vi "1553 Address Based Handles to Execution Unit Address Handles.vi"(8 "error in":errorcluster, 11 "1553 address based channel handles":T1[](array[typedef]) {"acyclic frame trigger handles"."handle" format="%.0x"; "start stop handles"."stop handle" format="%.0x"; "start stop handles"."start handle" format="%.0x"}) -> (0 "error out":errorcluster, 3 "address based channels":T4[](array[typedef]) format="%.0x")   [LabVIEW 2020, in "Ballard MIL-STD-1553 Engine.lvlib" / "Implementation.lvlib" / "Address Based Execution Unit.lvclass"]
uses:
  Address Based Execution Unit.lvclass
  <vilib>/NI VeriStand/Custom Device API/Custom Device Item Ref.ctl
  <vilib>/NI VeriStand/Custom Device API/Custom Device API.lvlib
  Shared/Address.ctl
  Start Stop Channel Handles.ctl
  1553 Address Based Handles.ctl
  Acyclic Frame Trigger Handle.ctl
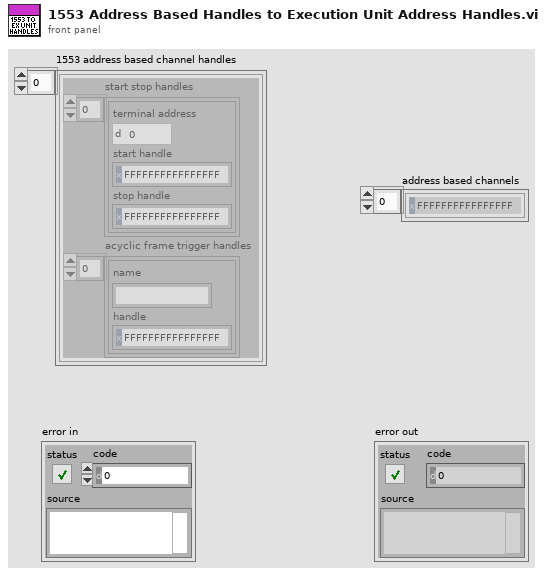
[diagram p1: front panel]
types:
  T1 = typedef "Ballard MIL-STD-1553 Engine.lvlib/Implementation.lvlib/Address Based Execution Unit.lvclass/1553 Address Based Handles.ctl" = cluster{"start stop handles":T2[], "acyclic frame trigger handles":T5[]}
  T2 = typedef "Ballard MIL-STD-1553 Engine.lvlib/Implementation.lvlib/Address Based Execution Unit.lvclass/Start Stop Channel Handles.ctl" = cluster{"terminal address":T3, "start handle":T4, "stop handle":T4}
  T3 = typedef "Address.ctl" = u16
  T4 = typedef "Custom Device API.lvlib/Custom Device Item Ref.ctl" = u64
  T5 = typedef "Ballard MIL-STD-1553 Engine.lvlib/Implementation.lvlib/Address Based Execution Unit.lvclass/Acyclic Frame Trigger Handle.ctl" = cluster{"name":string, "handle":T4}
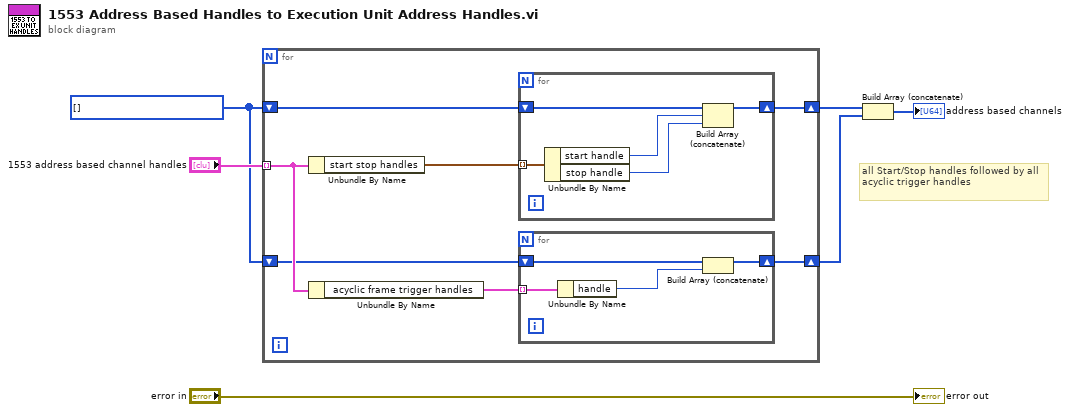
[diagram p0: block diagram]
diagram:
  w4 = T4[] [] ("Incoming Channels")
  # "all Start/Stop handles followed by all acyclic trigger handles"
  n1 = for {
    shift-right: [w9] -> w3
    shift-left: w4 -> [w13]
    tunnel: "1553 address based channel handles" -> [w10] mode=indexing
    shift-right: [w7] -> w1
    shift-left: w4 -> [w8]
    n2 = Unbundle By Name(w10) -> ("start stop handles"=w12:T2[])
    n3 = Unbundle By Name(w10) -> ("acyclic frame trigger handles"=w11:T5[])
    n4 = for {
      shift-right: [w21] -> w9
      shift-left: w13 -> [w22]
      tunnel: w12 -> [w20] mode=indexing
      n5 = Unbundle By Name(w20) -> ("start handle"=w19:T4, "stop handle"=w18:T4)
      n6 = Build Array (concatenate)(w22, w19, w18) -> (w21:T4[])
    }
    n7 = for {
      shift-right: [w16] -> w7
      shift-left: w8 -> [w17]
      tunnel: w11 -> [w15] mode=indexing
      n8 = Unbundle By Name(w15) -> ("handle"=w14:T4)
      n9 = Build Array (concatenate)(w17, w14) -> (w16:T4[])
    }
  }
  n10 = Build Array (concatenate)(w3, w1) -> (→"address based channels":T4[])
  "error out" <- "error in"
